vi "Configure Current.vi"(8 "Current（A）":dbl, 9 "error in (no error)":errorcluster, 10 "VISA resource name":refnum<visa-resource-name>) -> (1 "error out":errorcluster, 2 "VISA resource name out":refnum<visa-resource-name>)   [LabVIEW 2018]
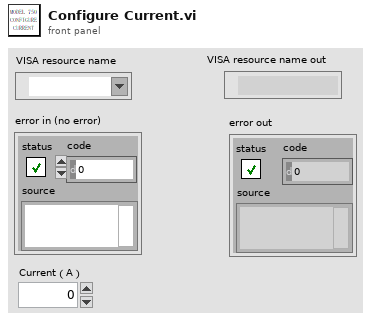
[diagram p1: front panel]
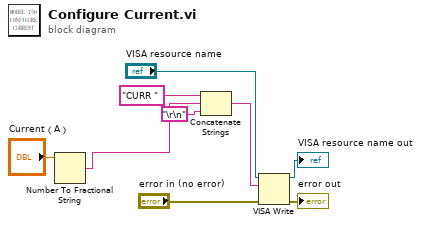
[diagram p0: block diagram]
diagram:
  n1 = Number To Fractional String(number="Current（A）") -> (F-format string=w2:string)  [unwired: 3 in]
  n2 = Concatenate Strings("CURR " ("字符串"), w2, "\r\n") -> (w6:string)
  n3 = VISA Write(VISA resource name="VISA resource name", write buffer=w6, error in (no error)="error in (no error)") -> (VISA resource name out=→"VISA resource name out":refnum<visa-resource-name>, error out=→"error out":errorcluster)  [unwired: 1 out]
